vi "create default alias.vi"(8 "error in":errorcluster, 11 "configuration in":refnum<class "SystemLink File configuration.lvclass">) -> (0 "error out":errorcluster, 2 "default alias":string, 3 "configuration out":refnum<class "SystemLink File configuration.lvclass">)   [LabVIEW 2015, in "SystemLink File configuration.lvclass"]
doc: "Copyright 2017 National Instruments Corporation\n\nLicensed under the Apache License, Version 2.0 (the \"License\"); you may not use this file except in compliance with the License. You may obtain a copy of the License at http://www.apache.org/licenses/LICENSE-2.0\nUnless required by applicable law or agreed to in writing, software distributed under the License is distributed on an \"AS IS\" BASIS, WITHOUT WARRANTIES OR CONDITIONS OF ANY KIND, either express or implied. See the License for the specific language governing permissions and limitations under the License."
uses:
  SystemLink File configuration.lvclass
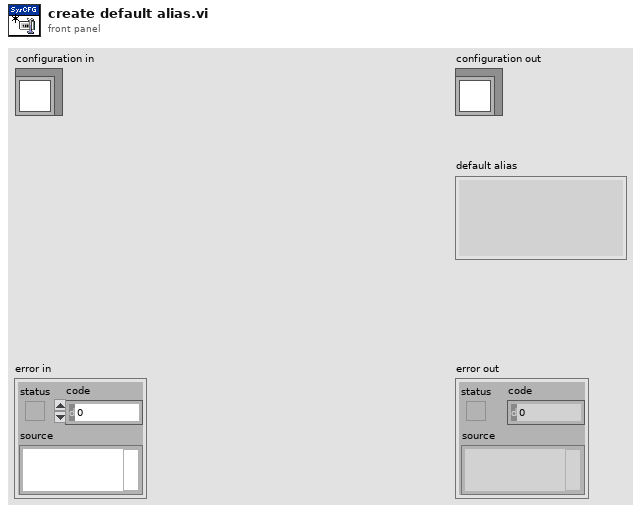
[diagram p1: front panel]
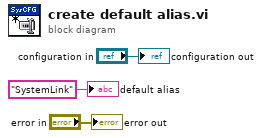
[diagram p0: block diagram]
diagram:
  "error out" <- "error in"
  "configuration out" <- "configuration in"
  "default alias" <- "SystemLink" ("default alias")
